vi "PH_Beamline.set 6P 4Q Position in GUI.vi"(0 "VI in":refnum<vi>, 2 "Index 6P 4Q Instance to change":i32, 5 "error in (no error)":errorcluster) -> (14 "VI out":refnum<vi>, 19 "error out":errorcluster)   [LabVIEW 2014, in "PH_Beamline.lvlib"]
uses:
  PH_Beamline.lvlib
  PH_BL-Master/PH_BL-Master.lvlib
  PH_Beamline_Common/PH_Beamline_Common.lvlib
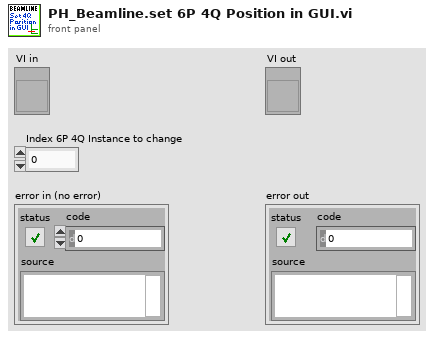
[diagram p1: front panel]
types:
  T1 = typedef "PH_BL-Master.lvlib/PH_BL-Master.i attribute.ctl" = cluster{"Remote controlled":bool, "Boolean Condition Service Subscriber":refnum<vi>[], "Picture Condition Service Subscriber":refnum<vi>[], "R2S":cluster{"GUI Ref":refnum<vi>, "State":bool}, "Vacua":cluster{"GUI Ref":refnum<vi>, "Limit":dbl, "Curr Value":dbl, "in range":bool}[], "O2 Inspection":cluster{"GUI Ref":refnum<vi>, "Concentration":dbl, "State":T2}[], "Boolean Status Service Subscriber":cluster{"GUI Ref":refnum<vi>, "Status":T2, "no Link?":bool, "Status Subscriber Class":T3}[], "Picture Status Service Subscriber":cluster{"GUI Ref":refnum<vi>, "Status":T2, "no Link?":bool, "Status Subscriber Class":T3}[], "6P 4Q Service Subscriber":cluster{"GUI Ref":refnum<vi>, "Selector":T4, "no Link?":bool}[], "Index of latest 6P 4Q changing Instance":i32, "Index of latest Picture Status changing Instance":i32, "Index of latest Boolean Status changing Instance":i32, "Vision ID on same Node":string, "Start Phase over?":bool, "GUI Ref Delete":refnum<vi>}
  T2 = typedef "PH_StatusHandler.lvlib/PH_StatusHandler.Status.ctl" = i16
  T3 = typedef "PH_BL-Master.lvlib/PH_BL-Master.Status Subscriber Class.ctl" = enum16{"unknown", "Switch", "BB", "6P Switch", "Switch GUI", "Switch and 6P State", "Force Sensor"}
  T4 = typedef "PH_4_Pos_Selector.lvlib/PH_4_Pos_Selector.Position Selector.ctl" = u16
  T5 = cluster{"GUI Ref":refnum<vi>, "Selector":T4, "no Link?":bool}[]
  T6 = cluster{"GUI Ref":refnum<vi>, "Selector":T4, "no Link?":bool}
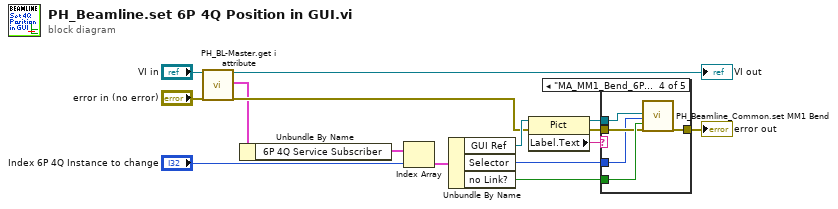
[diagram p0: block diagram]
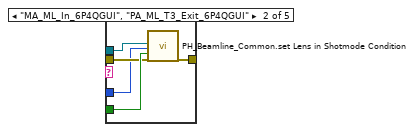
[diagram p3: hidden frame]
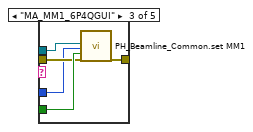
[diagram p4: hidden frame]
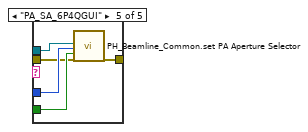
[diagram p5: hidden frame]
diagram:
  n1 = call "PH_BL-Master.get i attribute.vi"("i ref in"="VI in", "error in (no error)"="error in (no error)") -> ("i ref out"=→"VI out":refnum<vi>, "i attribute"=w4:T1, "error out"=w8:errorcluster)  [unwired: 15 in]
  n2 = Unbundle By Name(w4) -> ("6P 4Q Service Subscriber"=w5:T5)
  n3 = Index Array(array=w5, index="Index 6P 4Q Instance to change") -> (element=w7:T6)
  n4 = Unbundle By Name(w7) -> ("GUI Ref"=w9:refnum<vi>, "Selector"=w13:T4, "no Link?"=w14:bool)
  n5 = property class="Pict"(reference=w9, error in=w8) -> (reference out=w12:refnum<vi>, error out=w10:errorcluster, "Label.Text"=w15:string)
  n6 = case "Empty Strings" shown="\"MA_MM1_Bend_6P4QGUI\"" w15 {
    tunnel: w10 -> [w16 w19 w24 w29 w33]
    tunnel: w14 -> [_ w20 w25 w30 w35]
    tunnel: [w16 w21 w26 w31 w36] -> w11
    tunnel: w13 -> [_ w17 w22 w27 w34]
    tunnel: w12 -> [_ w18 w23 w28 w32]
    frame Default {
    }
    frame "MA_ML_In_6P4QGUI", "PA_ML_T3_Exit_6P4QGUI" {
      n7 = call "PH_Beamline_Common.set Lens in Shotmode Condition.vi"("CtlRef"=w18, "State"=w17, "no link"=w20, "error in (no error)"=w19) -> ("error out"=w21:errorcluster)  [unwired: 15 in]
    }
    frame "MA_MM1_6P4QGUI" {
      n8 = call "PH_Beamline_Common.set MM1.vi"("CtlRef"=w23, "State"=w22, "no link"=w25, "error in (no error)"=w24) -> ("error out"=w26:errorcluster)  [unwired: 15 in]
    }
    frame "MA_MM1_Bend_6P4QGUI" {
      n9 = call "PH_Beamline_Common.set MM1 Bend.vi"("CtlRef"=w28, "State"=w27, "no link"=w30, "error in (no error)"=w29) -> ("error out"=w31:errorcluster)  [unwired: 15 in]
    }
    frame "PA_SA_6P4QGUI" {
      n10 = call "PH_Beamline_Common.set PA Aperture Selector.vi"("CtlRef"=w32, "State"=w34, "no link"=w35, "error in (no error)"=w33) -> ("error out"=w36:errorcluster)  [unwired: 15 in]
    }
  }
  "error out" <- w11
